vi "Count2Indexes.vi"(1 "sweep_dim":u64[](array[numeric]), 2 "Count":u64) -> (0 "Indexes":u64[](array[numeric]))   [LabVIEW 2013]
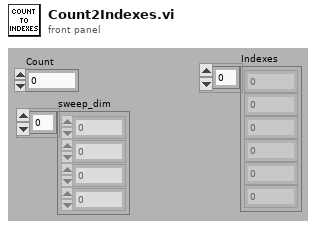
[diagram p1: front panel]
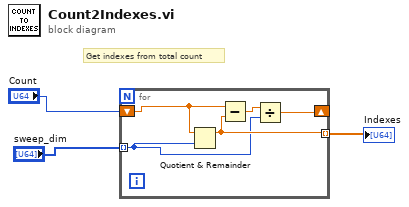
[diagram p0: block diagram]
diagram:
  # "Get indexes from total count"
  n1 = for {
    tunnel: "sweep_dim" -> [w4] mode=indexing
    tunnel: [w7] -> w2 mode=indexing
    shift-right: [w5] -> _
    shift-left: "Count" -> [w8]
    n2 = Quotient & Remainder(x=w8, y=w4) -> (x-y*floor(x/y)=w7:dbl)  [unwired: 1 out]
    n3 = Subtract(x=w8, y=w7) -> (x-y=w6:dbl)
    n4 = Divide(x=w6, y=w4) -> (x/y=w5:dbl)
  }
  "Indexes" <- w2
